vi "CAN Jaguar Heartbeat.vi"(8 "error in (no error)":errorcluster) -> (0 "error out":errorcluster)   [LabVIEW 2009, in "CAN.lvlib"]
uses:
  CAN.lvlib
  SubVIs/CAN System Message IDs.ctl
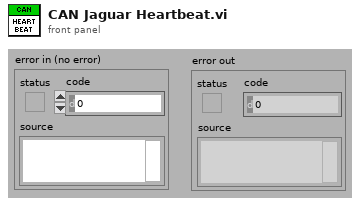
[diagram p1: front panel]
types:
  T1 = typedef "CAN.lvlib/CAN System Message IDs.ctl" = u32
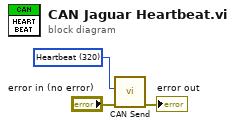
[diagram p0: block diagram]
diagram:
  w2 = T1 320 items=["Device Assignment"=128, "Device Query"=2147483840, "Sync Update"=384, "Firmware Update"=448, "Firmware Version"=2147484160, "Enumerate"=576, "Heartbeat"=320] ("CAN System Message IDs")
  n1 = call "CAN Send.vi"("error in (no error)"="error in (no error)", "messageID"=w2) -> ("error out"=→"error out":errorcluster)  [unwired: 1 in, 8 out]
